vi "plot grafici custom + tolleranze.vi"(6 "CURVE SINGOLE IN":T1, 7 "NM?":bool=TRUE, 8 "RENDIMENTI in":cluster{"X":dbl[], "Y":dbl[]}[](array[cluster]), 9 "CURVE IDRAULICHE in":cluster{"X":dbl[], "Y":dbl[]}[](array[cluster]), 10 "tolleranze":dbl[](array[numeric]) format="%#_6f %", 11 "grafici":dbl[][](array[numeric])) -> (0 "CURVE SINGOLE OUT":T1, 2 "RENDIMENTI":cluster{"X":dbl[], "Y":dbl[]}[](graph), 3 "CURVE IDRAULICHE":cluster{"X":dbl[], "Y":dbl[]}[](graph))   [LabVIEW 2019]
uses:
  TypeDef/Curve singole.ctl
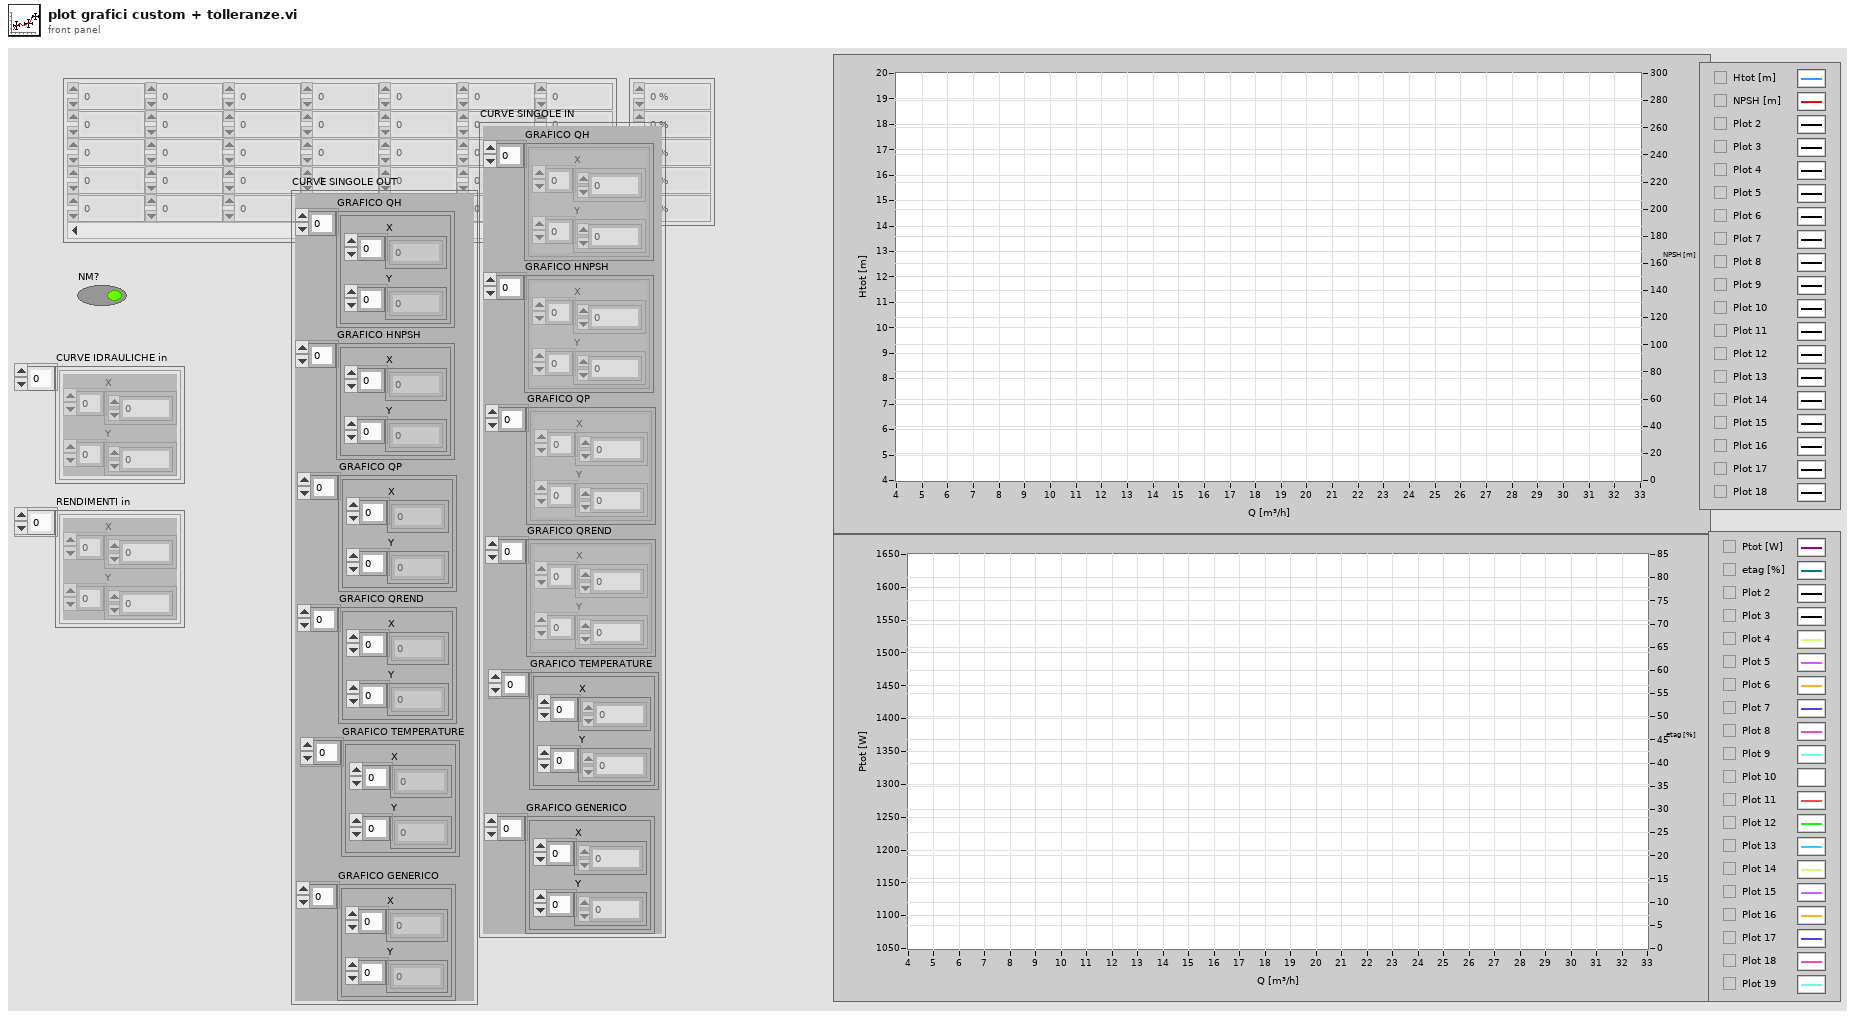
[diagram p1: front panel]
types:
  T1 = typedef "Curve singole.ctl" = cluster{"GRAFICO QH":cluster{"X":dbl[], "Y":dbl[]}[], "GRAFICO HNPSH":cluster{"X":dbl[], "Y":dbl[]}[], "GRAFICO QP":cluster{"X":dbl[], "Y":dbl[]}[], "GRAFICO QREND":cluster{"X":dbl[], "Y":dbl[]}[], "GRAFICO TEMPERATURE":cluster{"X":dbl[], "Y":dbl[]}[], "GRAFICO GENERICO":cluster{"X":dbl[], "Y":dbl[]}[]}
  T2 = cluster{"GRAFICO QNPSH":cluster{"X":dbl[], "Y":dbl[]}[], "GRAFICO QP":cluster{"X":dbl[], "Y":dbl[]}[], "GRAFICO QREND":cluster{"X":dbl[], "Y":dbl[]}[], "GRAFICO QH":cluster{"X":dbl[], "Y":dbl[]}[]}
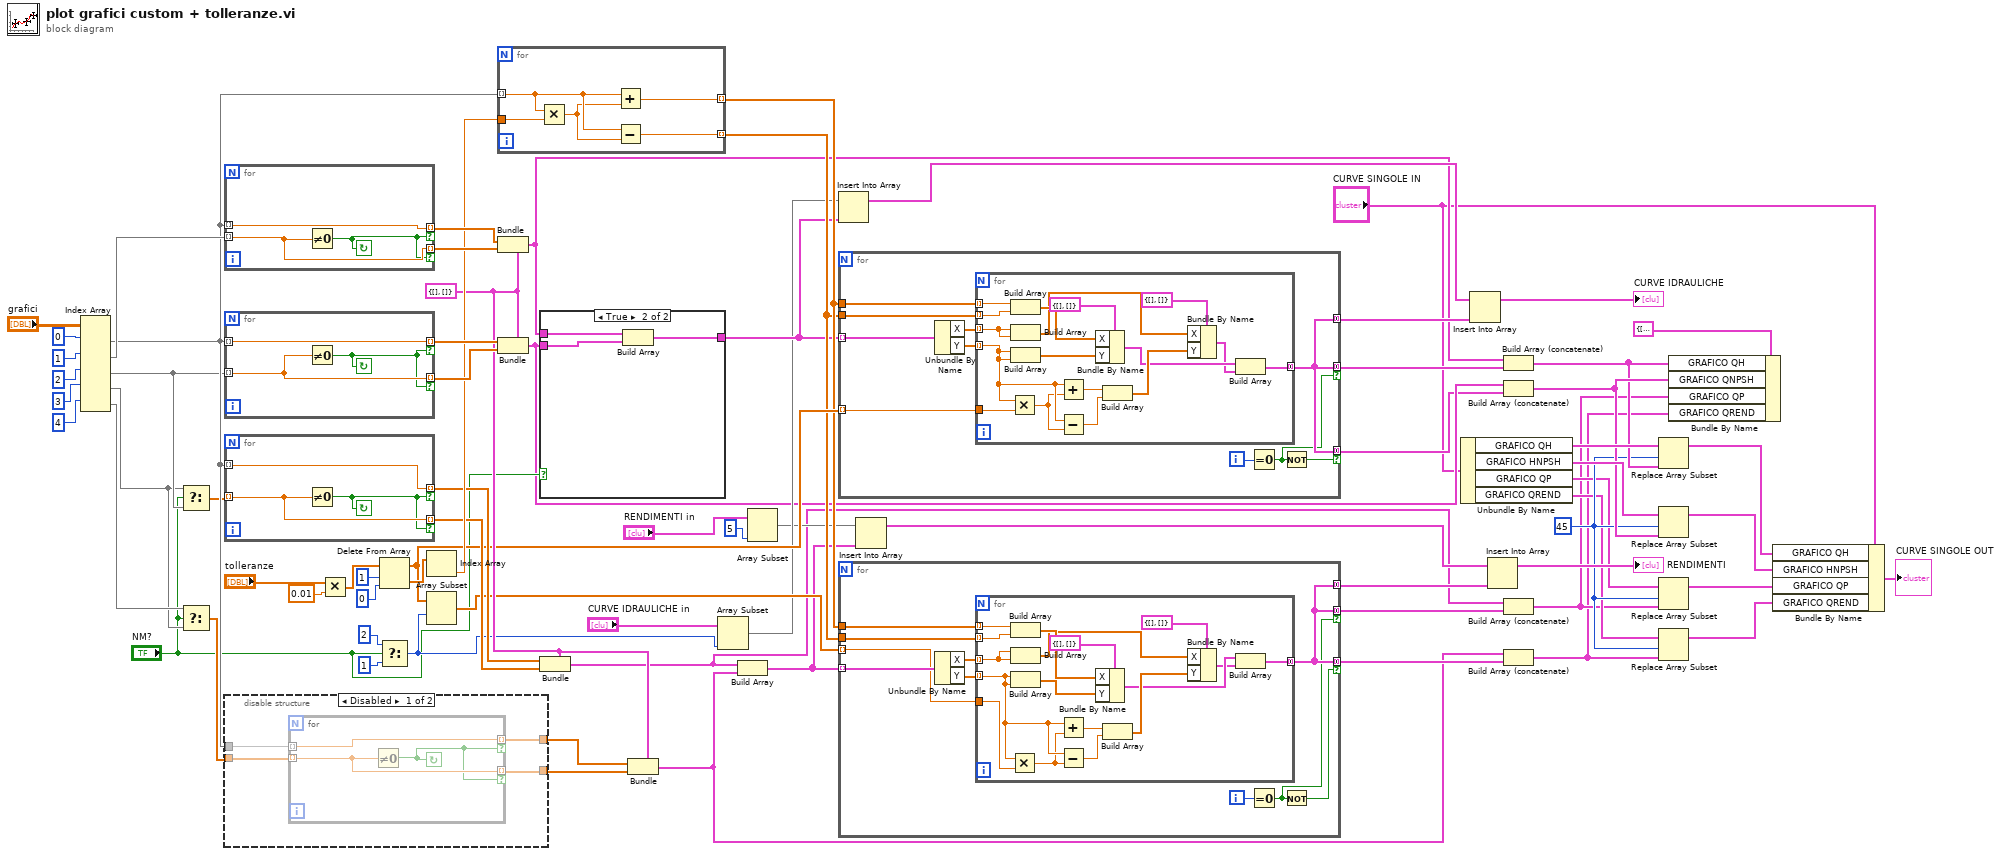
[diagram p0: block diagram]
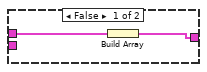
[diagram p3: hidden frame]
diagram:
  w9 = 45 ("index")
  w51 = cluster{"X":dbl[], "Y":dbl[]} {"X"=[], "Y"=[]} ("element")
  n1 = Index Array(array="grafici", index (row) #1=0 ("index (row)"), index (row) #2=1 ("index (row)"), index (row) #3=2 ("index (row)"), index (row) #4=3 ("disabled index (col)"), index (row) #5=4 ("index (row)")) -> (element #1=w54:dbl[], element #2=w70:dbl[], element #3=w32:dbl[], element #4=w29:dbl[], element #5=w30:dbl[])  [unwired: 5 in]
  n2 = Select(t=w29, s="NM?", f=w32) -> (s? t:f=w31:dbl[])
  n3 = Select(t=w30, s="NM?", f=w29) -> (s? t:f=w28:dbl[])
  n4 = for {
    tunnel: w70 -> [w77] mode=indexing
    tunnel: [w77] -> w69 mode=indexing if=w75
    tunnel: [w76] -> w68 mode=indexing if=w75
    tunnel: w54 -> [w76] mode=indexing
    stop <- w75 continue-if-true
    n5 = Not Equal To 0?(x=w77) -> (x != 0?=w75:bool)
  }
  n6 = for {
    tunnel: w32 -> [w80] mode=indexing
    tunnel: [w80] -> w66 mode=indexing if=w78
    tunnel: [w79] -> w67 mode=indexing if=w78
    tunnel: w54 -> [w79] mode=indexing
    stop <- w78 continue-if-true
    n7 = Not Equal To 0?(x=w80) -> (x != 0?=w78:bool)
  }
  n8 = for {
    tunnel: w31 -> [w83] mode=indexing
    tunnel: [w83] -> w52 mode=indexing if=w81
    tunnel: [w82] -> w53 mode=indexing if=w81
    tunnel: w54 -> [w82] mode=indexing
    stop <- w81 continue-if-true
    n9 = Not Equal To 0?(x=w83) -> (x != 0?=w81:bool)
  }
  n10 = disable-structure shown="Disabled" {
    disable-tunnel: w54 -> [w87 _]
    disable-tunnel: [w86 _] -> w50
    disable-tunnel: [w85 _] -> w49
    disable-tunnel: w28 -> [w84 _]
    frame Disabled {
      n11 = for {
        tunnel: w84 -> [w90] mode=indexing
        tunnel: [w90] -> w85 mode=indexing if=w88
        tunnel: [w89] -> w86 mode=indexing if=w88
        tunnel: w87 -> [w89] mode=indexing
        stop <- w88 continue-if-true
        n12 = Not Equal To 0?(x=w90) -> (x != 0?=w88:bool)
      }
    }
    frame Enabled {
    }
  }
  n13 = Multiply(x="tolleranze", y=0.01) -> (x*y=w58:dbl[])
  n14 = Delete From Array(array=w58, length=1, index=0) -> (deleted portion=w63:dbl[], array with subset deleted=w48:dbl[])
  n15 = Select(t=2 ("length"), s="NM?", f=1) -> (s? t:f=w27:i32)
  n16 = Index Array(array=w63) -> (element=w62:dbl)  [unwired: 1 in]
  n17 = Array Subset(array=w48, index=w27) -> (w47:dbl[])  [unwired: 1 in]
  n18 = for {
    tunnel: w54 -> [w94] mode=indexing
    tunnel: w62 -> [w95]
    tunnel: [w92] -> w46 mode=indexing
    tunnel: [w91] -> w45 mode=indexing
    n19 = Multiply(x=w94, y=w95) -> (x*y=w93:dbl)
    n20 = Add(x=w94, y=w93) -> (x+y=w92:dbl)
    n21 = Subtract(x=w94, y=w93) -> (x-y=w91:dbl)
  }
  n22 = Bundle(cluster=w51, "X"=w68, "Y"=w69) -> (w23:cluster{"X":dbl[], "Y":dbl[]})
  n23 = Bundle(cluster=w51, "X"=w67, "Y"=w66) -> (w21:cluster{"X":dbl[], "Y":dbl[]})
  n24 = case shown="True" "NM?" {
    tunnel: w21 -> [_ w100]
    tunnel: w23 -> [w97 w99]
    tunnel: [w96 w98] -> w43
    frame False {
      n25 = Build Array(w97) -> (w96:cluster{"X":dbl[], "Y":dbl[]}[])
    }
    frame True {
      n26 = Build Array(w99, w100) -> (w98:cluster{"X":dbl[], "Y":dbl[]}[])
    }
  }
  n27 = Bundle(cluster=w51, "X"=w53, "Y"=w52) -> (w18:cluster{"X":dbl[], "Y":dbl[]})
  n28 = Bundle(cluster=w51, "X"=w50, "Y"=w49) -> (w16:cluster{"X":dbl[], "Y":dbl[]})
  n29 = Array Subset "Array Subset"(array="CURVE IDRAULICHE in", length=w27) -> (w38:cluster{"X":dbl[], "Y":dbl[]}[])  [unwired: 1 in]
  n30 = Build Array(w18, w16) -> (w41:cluster{"X":dbl[], "Y":dbl[]}[])
  n31 = Array Subset(array="RENDIMENTI in", length=5) -> (w35:cluster{"X":dbl[], "Y":dbl[]}[])  [unwired: 1 in]
  n32 = Insert Into Array "Insert Into Array"(array=w38, new element=w43) -> (w42:cluster{"X":dbl[], "Y":dbl[]}[])  [unwired: 1 in]
  n33 = for {
    tunnel: w43 -> [w110] mode=indexing
    tunnel: w48 -> [w105] mode=indexing
    tunnel: w46 -> [w109]
    tunnel: w45 -> [w108]
    tunnel: [w104] -> w57 mode=concatenating
    tunnel: [w104] -> w22 mode=concatenating if=w102
    tunnel: [w104] -> w20 mode=concatenating if=w101
    i -> [w103]
    n34 = Unbundle By Name(w110) -> ("X"=w106:dbl[], "Y"=w107:dbl[])
    n35 = for {
      tunnel: w109 -> [w126] mode=indexing
      tunnel: w108 -> [w125] mode=indexing
      tunnel: w107 -> [w118] mode=indexing
      tunnel: w106 -> [w121] mode=indexing
      tunnel: w105 -> [w119]
      tunnel: [w111] -> w104 mode=concatenating
      n36 = Multiply(x=w118, y=w119) -> (x*y=w117:dbl)
      n37 = Build Array(w126, w125) -> (w124:dbl[])
      n38 = Build Array(w121, w121) -> (w120:dbl[])
      n39 = Build Array(w118, w118) -> (w123:dbl[])
      n40 = Add(x=w118, y=w117) -> (x+y=w116:dbl)
      n41 = Subtract(x=w118, y=w117) -> (x-y=w115:dbl)
      n42 = Bundle By Name(cluster=cluster{"X":dbl[], "Y":dbl[]} {"X"=[], "Y"=[]} ("element"), "X"=w124, "Y"=w123) -> (w113:cluster{"X":dbl[], "Y":dbl[]})
      n43 = Build Array(w116, w115) -> (w114:dbl[])
      n44 = Bundle By Name(cluster=cluster{"X":dbl[], "Y":dbl[]} {"X"=[], "Y"=[]} ("element"), "X"=w120, "Y"=w114) -> (w112:cluster{"X":dbl[], "Y":dbl[]})
      n45 = Build Array(w113, w112) -> (w111:cluster{"X":dbl[], "Y":dbl[]}[])
    }
    n46 = Equal To 0?(x=w103) -> (x = 0?=w102:bool)
    n47 = Not(x=w102) -> (.not. x?=w101:bool)
  }
  n48 = for {
    tunnel: w41 -> [w137] mode=indexing
    tunnel: w47 -> [w132] mode=indexing
    tunnel: w46 -> [w136]
    tunnel: w45 -> [w135]
    tunnel: [w130] -> w44 mode=concatenating
    tunnel: [w130] -> w19 mode=concatenating if=w129
    tunnel: [w130] -> w17 mode=concatenating if=w128
    i -> [w131]
    n49 = Unbundle By Name(w137) -> ("X"=w133:dbl[], "Y"=w134:dbl[])
    n50 = for {
      tunnel: w136 -> [w153] mode=indexing
      tunnel: w135 -> [w152] mode=indexing
      tunnel: w134 -> [w145] mode=indexing
      tunnel: w133 -> [w148] mode=indexing
      tunnel: w132 -> [w146]
      tunnel: [w138] -> w130 mode=concatenating
      n51 = Multiply(x=w145, y=w146) -> (x*y=w144:dbl)
      n52 = Build Array(w153, w152) -> (w151:dbl[])
      n53 = Build Array(w148, w148) -> (w147:dbl[])
      n54 = Build Array(w145, w145) -> (w150:dbl[])
      n55 = Add(x=w145, y=w144) -> (x+y=w143:dbl)
      n56 = Subtract(x=w145, y=w144) -> (x-y=w142:dbl)
      n57 = Bundle By Name(cluster=cluster{"X":dbl[], "Y":dbl[]} {"X"=[], "Y"=[]} ("element"), "X"=w151, "Y"=w150) -> (w140:cluster{"X":dbl[], "Y":dbl[]})
      n58 = Build Array(w143, w142) -> (w141:dbl[])
      n59 = Bundle By Name(cluster=cluster{"X":dbl[], "Y":dbl[]} {"X"=[], "Y"=[]} ("element"), "X"=w147, "Y"=w141) -> (w139:cluster{"X":dbl[], "Y":dbl[]})
      n60 = Build Array(w140, w139) -> (w138:cluster{"X":dbl[], "Y":dbl[]}[])
    }
    n61 = Equal To 0?(x=w131) -> (x = 0?=w129:bool)
    n62 = Not(x=w129) -> (.not. x?=w128:bool)
  }
  n63 = Insert Into Array(array=w35, new element=w41) -> (w40:cluster{"X":dbl[], "Y":dbl[]}[])  [unwired: 1 in]
  n64 = Unbundle By Name("CURVE SINGOLE IN") -> ("GRAFICO QH"=w14:cluster{"X":dbl[], "Y":dbl[]}[], "GRAFICO HNPSH"=w12:cluster{"X":dbl[], "Y":dbl[]}[], "GRAFICO QP"=w8:cluster{"X":dbl[], "Y":dbl[]}[], "GRAFICO QREND"=w7:cluster{"X":dbl[], "Y":dbl[]}[])
  n65 = Insert Into Array "Insert Into Array"(array=w42, new element=w57) -> (→"CURVE IDRAULICHE":cluster{"X":dbl[], "Y":dbl[]}[])  [unwired: 1 in]
  n66 = Insert Into Array(array=w40, new element=w44) -> (→"RENDIMENTI":cluster{"X":dbl[], "Y":dbl[]}[])  [unwired: 1 in]
  n67 = Build Array (concatenate)(w23, w22) -> (w10:cluster{"X":dbl[], "Y":dbl[]}[])
  n68 = Build Array (concatenate)(w21, w20) -> (w11:cluster{"X":dbl[], "Y":dbl[]}[])
  n69 = Build Array (concatenate)(w18, w19) -> (w3:cluster{"X":dbl[], "Y":dbl[]}[])
  n70 = Build Array (concatenate)(w16, w17) -> (w2:cluster{"X":dbl[], "Y":dbl[]}[])
  n71 = Replace Array Subset(array=w14, new element=w10, index=w9) -> (w13:cluster{"X":dbl[], "Y":dbl[]}[])
  n72 = Replace Array Subset(array=w12, new element=w11, index=w9) -> (w6:cluster{"X":dbl[], "Y":dbl[]}[])
  n73 = Replace Array Subset(array=w8, new element=w3, index=w9) -> (w5:cluster{"X":dbl[], "Y":dbl[]}[])
  n74 = Replace Array Subset(array=w7, new element=w2, index=w9) -> (w4:cluster{"X":dbl[], "Y":dbl[]}[])
  n75 = Bundle By Name(cluster=T2 {"GRAFICO QNPSH"=[], "GRAFICO QP"=[], "GRAFICO QREND"=[], "GRAFICO QH"=[]}, "GRAFICO QH"=w10, "GRAFICO QNPSH"=w11, "GRAFICO QP"=w3, "GRAFICO QREND"=w2) -> ()  [unwired: 1 out]
  n76 = Bundle By Name(cluster="CURVE SINGOLE IN", "GRAFICO QH"=w13, "GRAFICO HNPSH"=w6, "GRAFICO QP"=w5, "GRAFICO QREND"=w4) -> (→"CURVE SINGOLE OUT":T1)
